vi "Bind Formatted String.vi"(4 "Ignore Past Updates? (F)":bool, 5 "Datum Type":variant, 6 "Format String":string, 8 "error in (no error)":errorcluster, 9 "Datum Name (\"\"=Use Control Label)":string, 10 "Str Refnum":refnum<vi>, 11 "IViewable in":refnum<class "IViewable.lvclass">) -> (0 "error out":errorcluster, 3 "IViewable out":refnum<class "IViewable.lvclass">)   [LabVIEW 2017, in "IViewable.lvlib" / "IViewable.lvclass"]
doc: "Bind a string control terminal (control or indicator) to a published value. You must provide a format string that is valid for the specified datum type."
uses:
  IViewable.lvclass
  C:/Program Files (x86)/National Instruments/LabVIEW 2017/vi.lib/ActorFramework/Actor/Actor.lvclass
  <vilib>/ActorFramework/Actor/Actor.lvclass/Actor.ctl
  <vilib>/ActorFramework/Message Enqueuer/Message Enqueuer.lvclass/Message Enqueuer.ctl
  SubscriptionPolicy/ValueChangeSubscription/ValueChangeSubscription.lvclass/ValueChangeSubscription.ctl
  gpm_packages/@cs/transport/Source/Concrete/FormattedStringBinding/FormattedStringBinding.lvclass/FormattedStringBinding.ctl
  IMediator/SubscriptionRequest/SubscriptionRequest.lvclass/SubscriptionRequest.ctl
  IObserver/IObserver Messages/Subscribe Msg/Subscribe Msg.lvclass/Subscribe Msg.ctl
  <vilib>/ActorFramework/Message Enqueuer/Enqueue.vi
  <vilib>/ActorFramework/Message Enqueuer/Init from Existing Queue.vi
  SubscriptionPolicy/ValueChangeSubscription/ValueChangeSubscription.lvclass
  C:/Git/mva-framework/Source/Framework/IMediator/ISubscriptionPolicy/ISubscriptionPolicy.lvclass
  gpm_packages/@cs/transport/Source/Concrete/FormattedStringBinding/FormattedStringBinding.lvclass
  C:/Git/mva-framework/gpm_packages/@cs/transport/Source/Concrete/TerminalValueBinding/TerminalValueBinding.lvclass
  C:/Git/mva-framework/gpm_packages/@cs/transport/Source/ITransport/ITransport.lvclass
  IObserver/IObserver Messages/Subscribe Msg/Subscribe Msg.lvclass
  C:/Program Files (x86)/National Instruments/LabVIEW 2017/vi.lib/ActorFramework/Message/Message.lvclass
  <vilib>/ActorFramework/Message Priority Queue/Priority Enqueue.vi
  gpm_packages/@cs/transport/Source/Concrete/TerminalValueBinding/Construct Terminal Value Binding.vi
  <vilib>/Utility/error.llb/Error Cluster From Error Code.vi
  <vilib>/ActorFramework/Message Enqueuer/Message Enqueuer.lvclass
  IMediator/SubscriptionRequest/SubscriptionRequest.lvclass
  <vilib>/ActorFramework/Actor/Actor.lvclass
  IMediator/ISubscriptionPolicy/ISubscriptionPolicy.lvclass
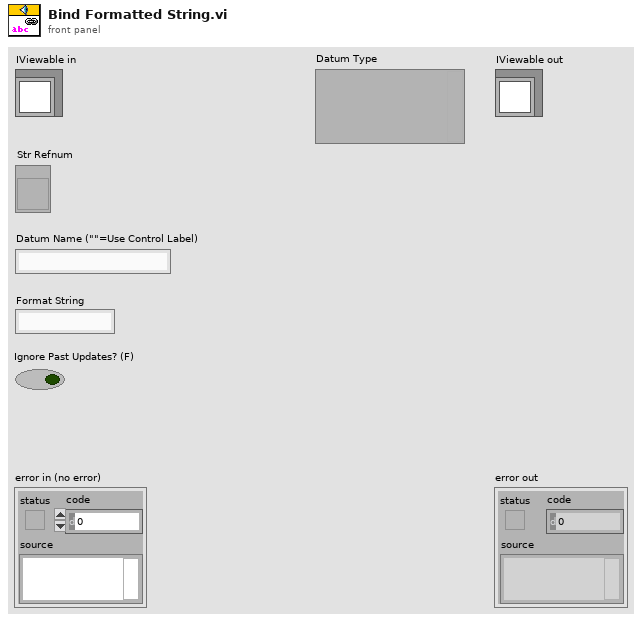
[diagram p1: front panel]
types:
  T1 = typedef "IMediator.lvlib/ISubscriptionPolicy.lvclass/ISubscriptionPolicy Reference.ctl" = refnum<data-value>
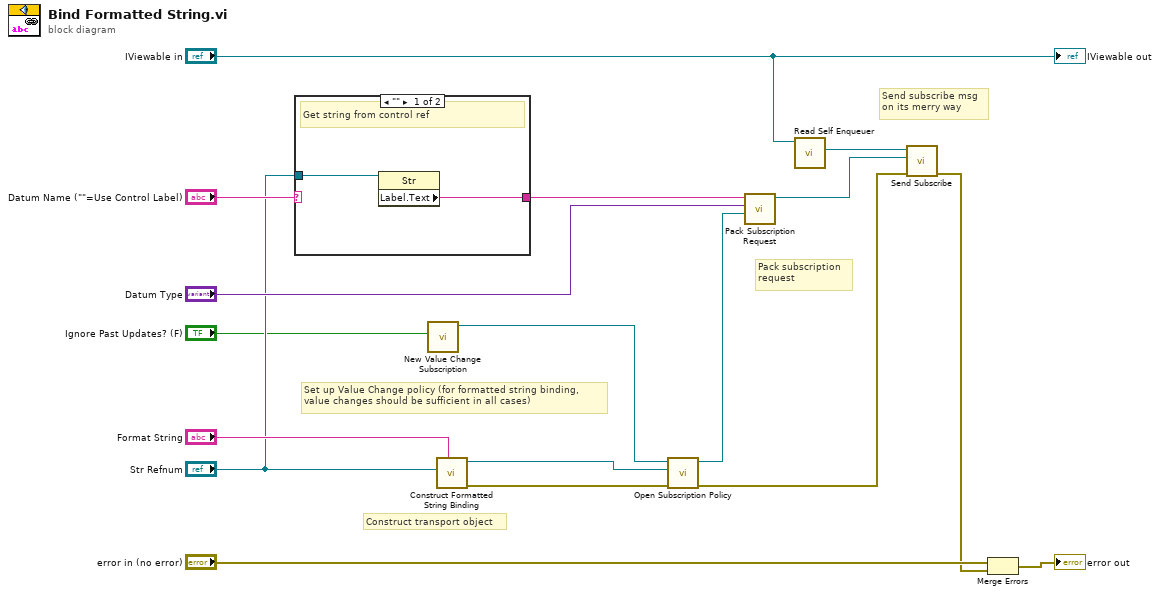
[diagram p0: block diagram]
diagram:
  # "Set up Value Change policy (for formatted string binding,\nvalue changes should be sufficient in all cases)"
  # "Send subscribe msg\non its merry way"
  # "Pack subscription\nrequest"
  # "Construct transport object"
  n1 = case shown="\"\"" "Datum Name (\"\"=Use Control Label)" {
    selector: "Datum Name (\"\"=Use Control Label)" -> [_ w20]
    tunnel: [w18 w20] -> w11
    tunnel: "Str Refnum" -> [w19 _]
    frame "" {
      # "Get string from control ref"
      n2 = property class="Str"(reference=w19) -> ("Label.Text"=w18:string)  [unwired: 1 in, 2 out]
    }
    frame Default {
      # "Use string wired to input terminal"
    }
  }
  n3 = call "New Value Change Subscription.vi"("Ignore Past Updates? (F)"="Ignore Past Updates? (F)") -> ("ValueChangeSubscription Out"=w4:refnum<class "ValueChangeSubscription.lvclass">)  [unwired: 10 in]
  n4 = call "Construct Formatted String Binding.vi"("Format String"="Format String", "Str Refnum"="Str Refnum") -> ("error out"=w2:errorcluster, "FormattedStringBinding"=w7:refnum<class "FormattedStringBinding.lvclass">)  [unwired: 8 in]
  n5 = call "Open Subscription Policy.vi"("error in (no error)"=w2, "Transport"=w7, "SubscriptionPolicy"=w4) -> ("error out"=w1:errorcluster, "Subscription Policy"=w3:T1)  [unwired: 7 in]
  n6 = call "Pack Subscription Request.vi"("Subscription Policy"=w3, "Type"="Datum Type", "Datum Name"=w11) -> ("SubscriptionRequest"=w6:refnum<class "SubscriptionRequest.lvclass">)  [unwired: 8 in]
  n7 = call <vilib>:"Read Self Enqueuer.vi"("Actor"="IViewable in") -> ("Self Enqueuer"=w15:refnum<class "Message Enqueuer.lvclass">)  [unwired: 10 in]
  n8 = call "Send Subscribe.vi"("error in (no error)"=w1, "SubscriptionRequest"=w6, "Message Enqueuer"=w15) -> ("error out"=w13:errorcluster)  [unwired: 7 in, 1 out]
  n9 = Merge Errors("error in (no error)", w13) -> (→"error out":errorcluster)
  "IViewable out" <- "IViewable in"
